vi "Set Window Pos.vi"(8 "error in (no error)":errorcluster, 10 "Front Panel Window:Panel Bounds":T1, 11 "Philosopher in":refnum<class "Philosopher.lvclass">) -> (0 "error out":errorcluster, 3 "Philosopher out":refnum<class "Philosopher.lvclass">)   [LabVIEW 2023, in "Philosopher.lvlib" / "Philosopher.lvclass"]
uses:
  Philosopher.lvclass
  <vilib>/Utility/miscctls.llb/LVRectTypeDef.ctl
  Philosopher.lvclass/Philosopher.ctl
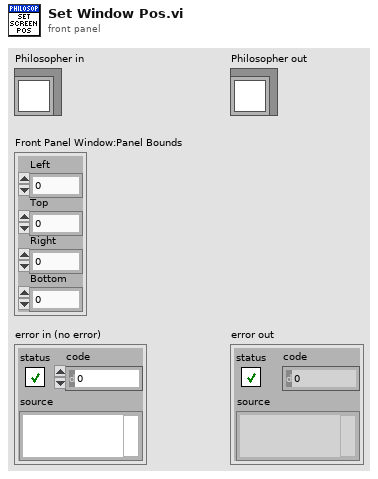
[diagram p1: front panel]
types:
  T1 = typedef "LVRectTypeDef.ctl" = cluster{"Left":i16, "Top":i16, "Right":i16, "Bottom":i16}
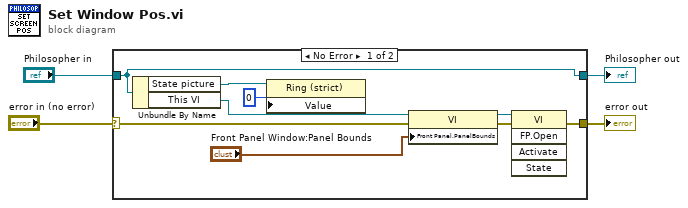
[diagram p0: block diagram]
diagram:
  n1 = case shown="No Error" "error in (no error)" {
    selector: "error in (no error)" -> [w13 w15]
    tunnel: [w9 w15] -> w3
    tunnel: [w12 w14] -> w1
    tunnel: "Philosopher in" -> [w12 w14]
    frame No Error {
      n2 = Unbundle By Name(w12) -> ("State picture"=w6:refnum<vi>, "This VI"=w11:refnum<vi>)
      n3 = property class="Ring (strict)"(reference=w6, "Value"=u16 0) -> ()  [unwired: 1 in, 2 out]
      n4 = property class="VI"(reference=w11, error in=w13, "Front Panel.PanelBounds"="Front Panel Window:Panel Bounds") -> (reference out=w7:refnum<vi>, error out=w8:errorcluster)
      n5 = invoke class="VI" method="FP.Open"(reference=w7, error in=w8) -> (error out=w9:errorcluster)  [unwired: 3 in, 4 out]
    }
    frame Error {
    }
  }
  "error out" <- w3
  "Philosopher out" <- w1
